vi "LVObject to JSON - Error in To JSON - Returns Error.vi"() -> ()   [LabVIEW 2017, in "JSON Serializable Serializer Tests.lvlib"]
uses:
  JSON Serializable Serializer Tests.lvlib
  JSON Serializable Serializer/JSON Serializable Serializer.lvclass
  <vilib>/Utility/error.llb/Error Cluster From Error Code.vi
  <vilib>/addons/_JKI Toolkits/Caraya/classes/Assert/Assert Error.vi
  <vilib>/ErrorRing/Error Ring.xnode
  <vilib>/addons/_JKI Toolkits/Caraya/classes/Test/Test.lvclass
  <vilib>/addons/_JKI Toolkits/Caraya/classes/Assert/Assert.lvclass
  Mock JSON Serializable/Mock JSON Serializable.lvclass
panel:
  out "error out":errorcluster
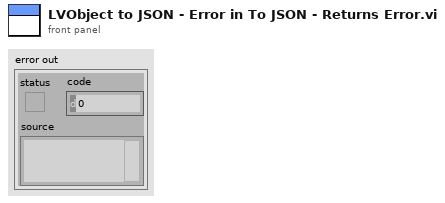
[diagram p1: front panel]
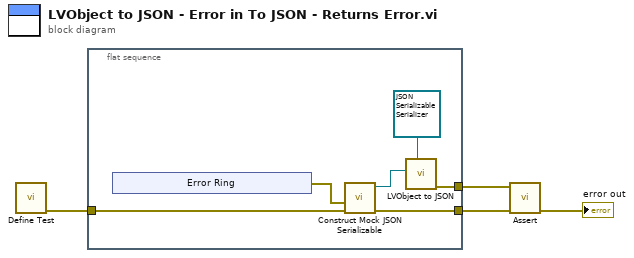
[diagram p0: block diagram]
diagram:
  n1 = call <vilib>:"Define Test.vi"() -> ("error out"=w3:errorcluster)  [unwired: 11 in]
  n2 = flat-sequence {
    tunnel: [w8] -> w4
    tunnel: w3 -> [w7]
    tunnel: [w9] -> w1
    frame #0 {
      n3 = xnode "Error Ring"() -> ("error out"=w5:errorcluster)
      n4 = call "Construct Mock JSON Serializable.vi"("error in (no error)"=w7, "From/To JSON <error out> (no error)"=w5) -> ("error out"=w8:errorcluster, "Mock JSON Serializable"=w6:refnum<class "Mock JSON Serializable.lvclass">)  [unwired: 8 in]
      n5 = call-dynamic "LVObject to JSON.vi"("JSON Serializer in"=refnum<class "JSON Serializable Serializer.lvclass"> refnum ("JSON Serializer.lvclass"), "Object"=w6) -> ("error out"=w9:errorcluster)  [unwired: 8 in, 1 out]
    }
  }
  n6 = call-poly <vilib>:"Assert.vi"("error in (no error)"=w4, "Error?"=w1) -> ("error out"=→"error out":errorcluster)  [unwired: 9 in]
